vi "Comparizon6.vi"() -> ()   [LabVIEW 2023]
panel:
  in  "Poppins Black Italic 18pt (W:900) 2":string="The quick brown fox jumps over the lazy dog 1234567890"
  in  "Poppins Black 18pt (W:900) 2":string="The quick brown fox jumps over the lazy dog 1234567890"
  in  "Poppins Extra Bold Italic 18pt (W:800) 2":string="The quick brown fox jumps over the lazy dog 1234567890"
  in  "Poppins Extra Bold 18pt (W:800) 2":string="The quick brown fox jumps over the lazy dog 1234567890"
  in  "Poppins Bold Italic18pt (W:700) 2":string="The quick brown fox jumps over the lazy dog 1234567890"
  in  "Poppins Bold 18pt (W:700) 2":string="The quick brown fox jumps over the lazy dog 1234567890"
  in  "Poppins Semi Bold Italic 18pt (W:650) 2":string="The quick brown fox jumps over the lazy dog 1234567890"
  in  "Poppins Semi Bold 18pt (W:600) 2":string="The quick brown fox jumps over the lazy dog 1234567890"
  in  "Poppins Italic 18pt (W:400) 2":string="The quick brown fox jumps over the lazy dog 1234567890"
  in  "Poppins Regular 18pt (W:400) 2":string="The quick brown fox jumps over the lazy dog 1234567890"
  in  "Poppins Medium Italic 18pt (W:500) 2":string="The quick brown fox jumps over the lazy dog 1234567890"
  in  "Poppins Medium 18pt (W:500) 2":string="The quick brown fox jumps over the lazy dog 1234567890"
  in  "Poppins Extra Light Italic 18pt (W:275) 2":string="The quick brown fox jumps over the lazy dog 1234567890"
  in  "Poppins Extra Light 18pt (W:275) 2":string="The quick brown fox jumps over the lazy dog 1234567890"
  in  "Poppins Thin Italic 18pt (Weight 250) 2":string="The quick brown fox jumps over the lazy dog 1234567890"
  in  "Poppins Thin 18pt (W:250) 2":string="The quick brown fox jumps over the lazy dog 1234567890"
  in  "Poppins Light Italic 18pt (W:300) 2":string="The quick brown fox jumps over the lazy dog 1234567890"
  in  "Poppins Light 18pt (W:300) 2":string="The quick brown fox jumps over the lazy dog 1234567890"
  in  "Segoe UI Black Italic 15pt (W:900)":string="The quick brown fox jumps over the lazy dog 1234567890 1111"
  in  "Segoe UI Black15pt (W:900)":string="The quick brown fox jumps over the lazy dog 1234567890 1111"
  in  "Segoe UI Bold Italic15pt (W:700)":string="The quick brown fox jumps over the lazy dog 1234567890 1111"
  in  "Segoe UI Bold 15pt (W:700)":string="The quick brown fox jumps over the lazy dog 1234567890 1111"
  in  "Segoe UI Semi Bold Italic15pt (W:600)":string="The quick brown fox jumps over the lazy dog 1234567890 1111"
  in  "Segoe UI Semi Bold 15pt (W:600)":string="The quick brown fox jumps over the lazy dog 1234567890 1111"
  in  "Segoe UI Italic15pt (W:400)":string="The quick brown fox jumps over the lazy dog 1234567890 1111"
  in  "Segoe UI 15pt (W:400)":string="The quick brown fox jumps over the lazy dog 1234567890 1111"
  in  "Segoe UI Semi Light Italic15pt (W:350)":string="The quick brown fox jumps over the lazy dog 1234567890 1111"
  in  "Segoe UI Semi Light 15pt (W:350)":string="The quick brown fox jumps over the lazy dog 1234567890 1111"
  in  "Segoe UI Ligt Italic15pt (W:300)":string="The quick brown fox jumps over the lazy dog 1234567890 1111"
  in  "Segoe UI Light 15pt (W:300)":string="The quick brown fox jumps over the lazy dog 1234567890 1111"
  in  "Poppins Thin Italic 18pt (Weight 250)":string="The quick brown fox jumps over the lazy dog 1234567890"
  in  "Poppins Thin 18pt (W:250)":string="The quick brown fox jumps over the lazy dog 1234567890"
  in  "Poppins Semi Bold Italic 18pt (W:650)":string="The quick brown fox jumps over the lazy dog 1234567890"
  in  "Poppins Semi Bold 18pt (W:600)":string="The quick brown fox jumps over the lazy dog 1234567890"
  in  "Poppins Regular 18pt (W:400)":string="The quick brown fox jumps over the lazy dog 1234567890"
  in  "Poppins Medium Italic 18pt (W:500)":string="The quick brown fox jumps over the lazy dog 1234567890"
  in  "Poppins Medium 18pt (W:500)":string="The quick brown fox jumps over the lazy dog 1234567890"
  in  "Poppins Light Italic 18pt (W:300)":string="The quick brown fox jumps over the lazy dog 1234567890"
  in  "Poppins Light 18pt (W:300)":string="The quick brown fox jumps over the lazy dog 1234567890"
  in  "Poppins Italic 18pt (W:400)":string="The quick brown fox jumps over the lazy dog 1234567890"
  in  "Poppins Extra Light Italic 18pt (W:275)":string="The quick brown fox jumps over the lazy dog 1234567890"
  in  "Poppins Extra Light 18pt (W:275)":string="The quick brown fox jumps over the lazy dog 1234567890"
  in  "Poppins Extra Bold Italic 18pt (W:800)":string="The quick brown fox jumps over the lazy dog 1234567890"
  in  "Poppins Extra Bold 18pt (W:800)":string="The quick brown fox jumps over the lazy dog 1234567890"
  in  "Poppins Bold Italic18pt (W:700)":string="The quick brown fox jumps over the lazy dog 1234567890"
  in  "Poppins Bold 18pt (W:700)":string="The quick brown fox jumps over the lazy dog 1234567890"
  in  "Poppins Black Italic 18pt (W:900)":string="The quick brown fox jumps over the lazy dog 1234567890"
  in  "Poppins Black 18pt (W:900)":string="The quick brown fox jumps over the lazy dog 1234567890"
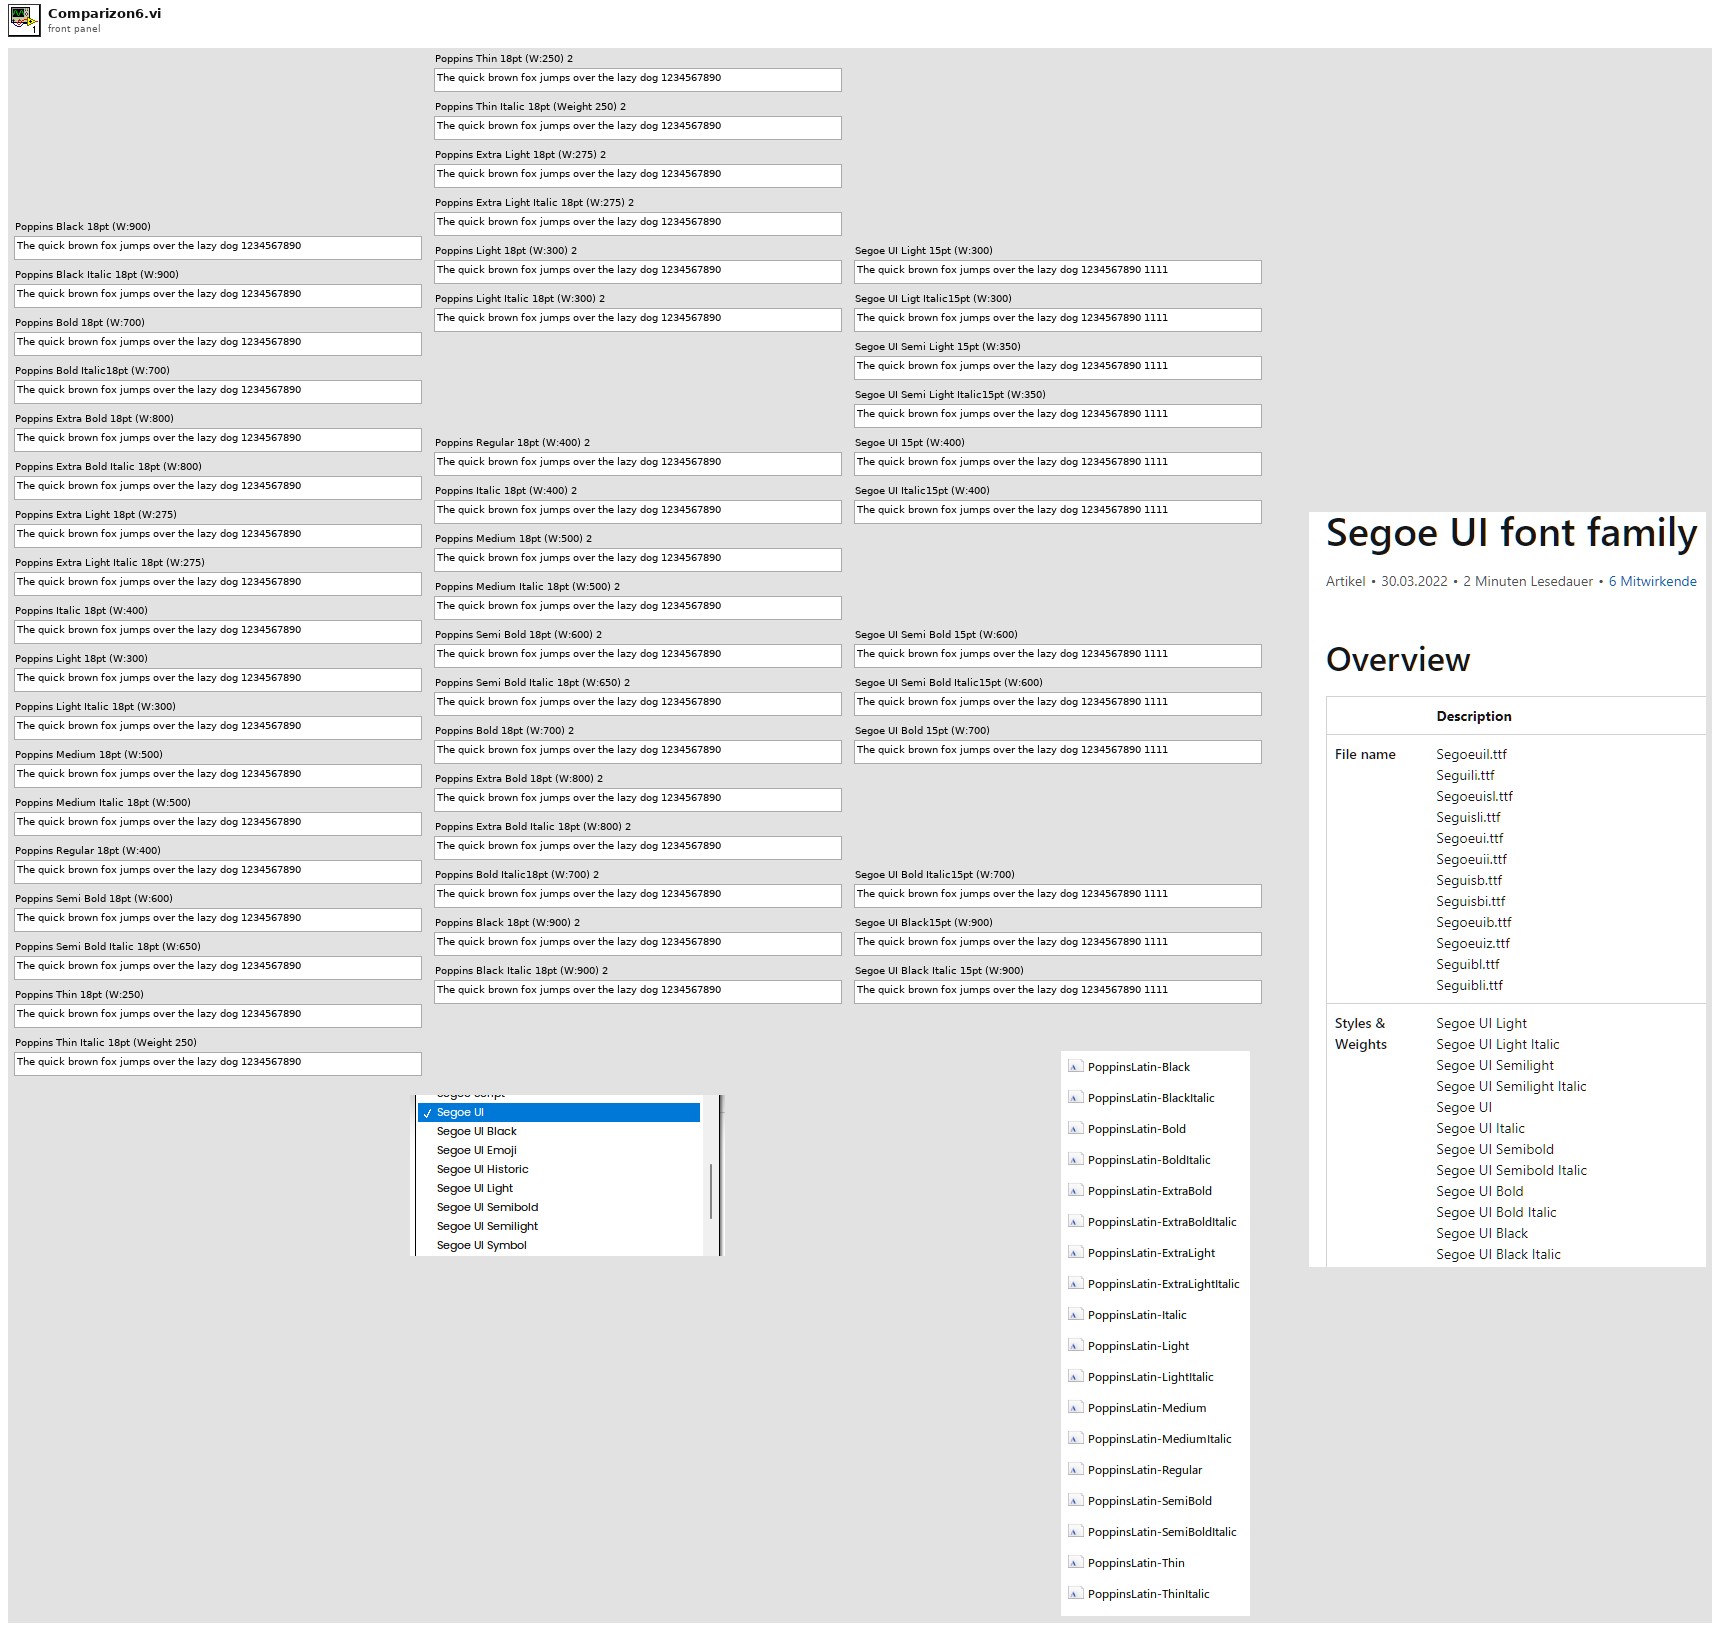
[diagram p1: front panel]
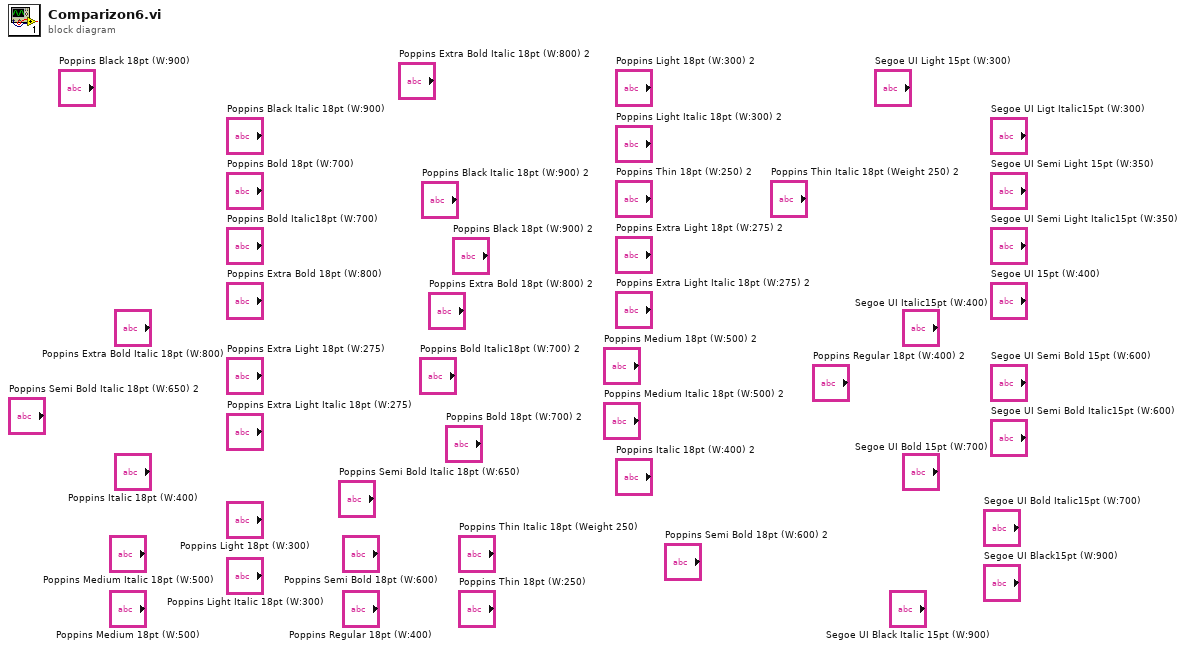
[diagram p0: block diagram]
diagram:
